vi "Signal Processing - Correct direction.vi"(8 "Correct":bool=TRUE, 10 "Right":i32, 11 "Left":i32) -> (0 "Reward":i32, 1 "Right":bool, 2 "Wrong":bool=TRUE, 3 "No response":bool)   [LabVIEW 2010, in "Core SubVIs.lvlib"]
uses:
  Core SubVIs.lvlib
panel:
  in  "Down":i32
  in  "Up":i32
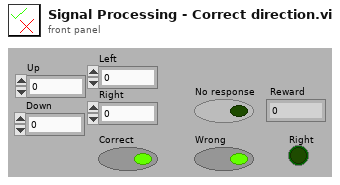
[diagram p1: front panel]
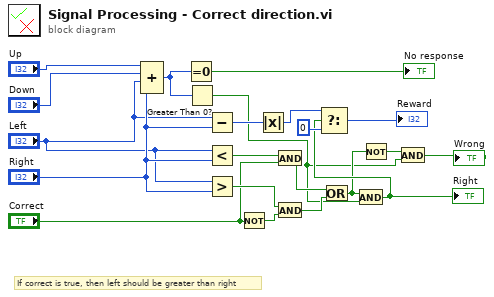
[diagram p0: block diagram]
diagram:
  # "If correct is true, then left should be greater than right"
  n1 = Compound Arithmetic op=ADD("Up", "Down", "Left", "Right") -> (w6:i32)
  n2 = Equal To 0?(x=w6) -> (x = 0?=→"No response":bool)
  n3 = Greater Than 0?(x=w6) -> (x > 0?=w2:bool)
  n4 = Subtract(x="Left", y="Right") -> (x-y=w19:i32)
  n5 = Less?(x="Left", y="Right") -> (x < y?=w13:bool)
  n6 = Greater?(x="Left", y="Right") -> (0:w14:bool)
  n7 = Not(x="Correct") -> (.not. x?=w8:bool)
  n8 = Absolute Value(x=w19) -> (abs(x)=w10:i32)
  n9 = And(x=w13, y="Correct") -> (x .and. y?=w11:bool)
  n10 = And(x=w14, y=w8) -> (x .and. y?=w12:bool)
  n11 = Or(x=w11, y=w12) -> (x .or. y?=w4:bool)
  n12 = And(x=w4, y=w2) -> (x .and. y?=w5:bool)
  "Right" <- w5
  n13 = Select(t=w10, s=w5, f=0) -> (s? t:f=→"Reward":i32)
  n14 = Not(x=w4) -> (.not. x?=w3:bool)
  n15 = And(x=w3, y=w2) -> (x .and. y?=→"Wrong":bool)
